vi "Dev Mode.vi"() -> (0 "Dev Mode":bool)   [LabVIEW 2022 SP3, in "FlexBlocks Support.lvlib"]
uses:
  FlexBlocks Support.lvlib
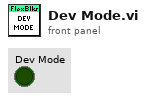
[diagram p1: front panel]
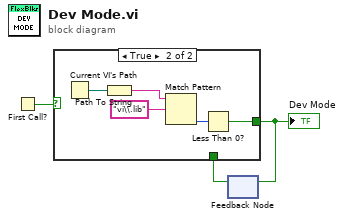
[diagram p0: block diagram]
diagram:
  n1 = First Call?() -> (First Call?: T/F=w3:bool)
  n2 = feedback #1() -> (w1:bool)  [unwired: 1 in]
  n3 = case shown="True" w3 {
    tunnel: [w4 w5] -> w2
    tunnel: w1 -> [w4 _]
    frame False {
    }
    frame True {
      n4 = Current VI's Path() -> (path=w9:path)
      n5 = Path To String(path=w9) -> (string=w8:string)
      n6 = Match Pattern(string=w8, regular expression="vi\\.lib") -> (offset past match=w6:i32)  [unwired: 1 in, 3 out]
      n7 = Less Than 0?(x=w6) -> (x < 0?=w5:bool)
    }
  }
  "Dev Mode" <- w2
  n8 = feedback-in #1(w2) -> ()
